vi "FPGA Read FFT.vi"(8 "error in (no error)":errorcluster) -> (0 "error out":errorcluster, 3 "Spectral Information":dbl[](array[numeric]))   [LabVIEW 2017]
uses:
  FPGA Global Variables.vi
  <vilib>/Utility/error.llb/Error Cluster From Error Code.vi
  <vilib>/rvi/errors/niLvFpgaAdjustHostInterfaceError.vi
  <vilib>/rvi/interface/nirviMethod/nirviMethod.xnode
  <vilib>/FPGAPlugInAG/Dynamic/niLvFpga_ReadFifo_Dynamic.vi
  <vilib>/rvi/errors/niLvFpgaMergeErrorWithErrorCode.vi
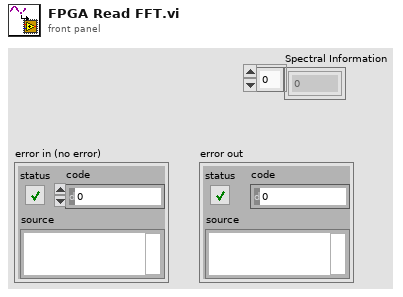
[diagram p1: front panel]
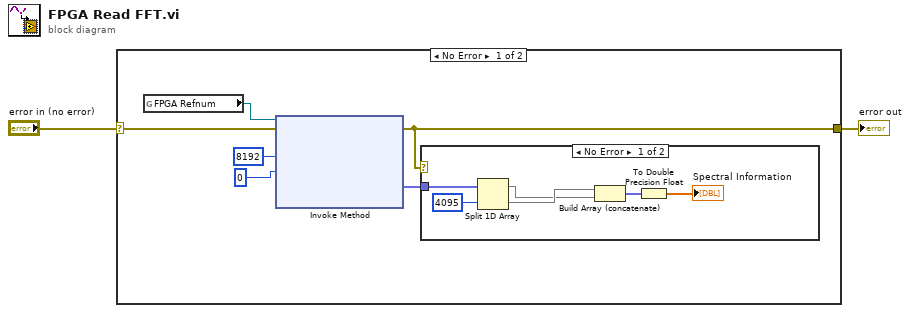
[diagram p0: block diagram]
diagram:
  n1 = case shown="No Error" "error in (no error)" {
    selector: "error in (no error)" -> [w5 w15]
    tunnel: [w3 w15] -> w2
    frame No Error {
      n2 = global read "FPGA Global Variables.vi" "FPGA Refnum"() -> (w8:refnum<k20>)
      n3 = xnode "Invoke Method"("FPGA VI Reference In"=w8, "error in"=w5, "Number of Elements"=u32 8192, "Timeout (ms)"=0) -> ("error out"=w3:errorcluster, "Data"=w4:fxp<+,32,5>[])  [unwired: 2 out]
      n4 = case shown="No Error" w3 {
        tunnel: w4 -> [w11 _]
        frame No Error {
          n5 = Split 1D Array(array=w11, index=4095) -> (first subarray=w9:fxp<+,32,5>[], second subarray=w13:fxp<+,32,5>[])
          n6 = Build Array (concatenate)(w13, w9) -> (w14:fxp<+,32,5>[])
          n7 = To Double Precision Float(number=w14) -> (double precision float=→"Spectral Information":dbl[])
        }
        frame Error {
        }
      }
    }
    frame Error {
    }
  }
  "error out" <- w2
